vi "sub_process data.vi"(0 "Processed Queue in":refnum<queue>, 1 "Elapsed Time (s)":dbl, 5 "Processed error in":errorcluster, 9 "Raw Queue in":refnum<queue>, 11 "Raw error in":errorcluster, 12 "Raw Data in":dbl[](array[numeric])) -> (4 "Processed Queue out":refnum<queue>, 6 "Processed error out":errorcluster, 10 "Raw Queue out":refnum<queue>, 14 "Processed Data Out":dbl[](array[numeric]), 15 "Raw error out":errorcluster)   [LabVIEW 2021]
uses:
  globalvariables.vi
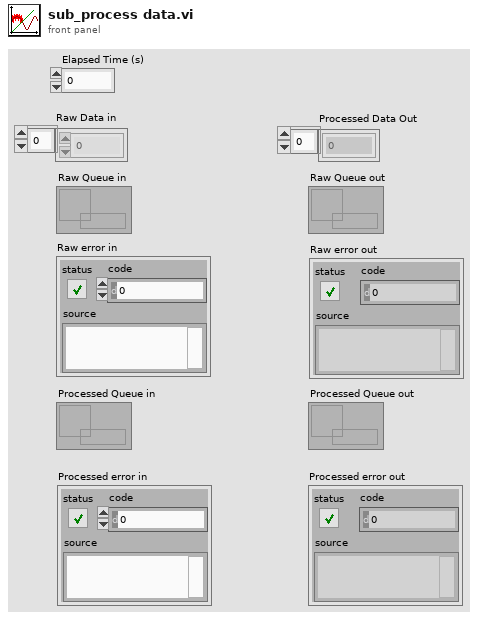
[diagram p1: front panel]
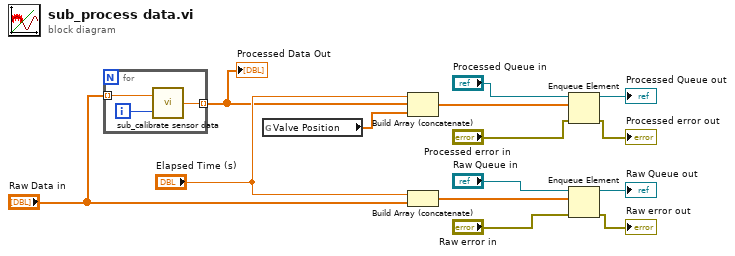
[diagram p0: block diagram]
diagram:
  n1 = for {
    tunnel: "Raw Data in" -> [w16] mode=indexing
    tunnel: [w15] -> w2 mode=indexing
    i -> [w17]
    n2 = call "sub_calibrate sensor data.vi"("Sensor Column"=w17, "Raw Data"=w16) -> ("Calibrated Data"=w15:dbl)
  }
  "Processed Data Out" <- w2
  n3 = global read "globalvariables.vi" "Valve Position"() -> (w1:dbl[])
  n4 = Build Array (concatenate)("Elapsed Time (s)", w2, w1) -> (w4:dbl[])
  n5 = Build Array (concatenate)("Elapsed Time (s)", "Raw Data in") -> (w13:dbl[])
  n6 = Enqueue Element(queue="Processed Queue in", element=w4, error in (no error)="Processed error in") -> (queue out=→"Processed Queue out":refnum<queue>, error out=→"Processed error out":errorcluster)  [unwired: 1 in, 1 out]
  n7 = Enqueue Element(queue="Raw Queue in", element=w13, error in (no error)="Raw error in") -> (queue out=→"Raw Queue out":refnum<queue>, error out=→"Raw error out":errorcluster)  [unwired: 1 in, 1 out]
